vi "TBQ_AddPoint.vi"(9 "New Data Point":dbl, 11 "TimeBasedQueue In":refnum<class "TimeBasedQueue.lvclass">) -> (3 "TimeBasedQueue Out":refnum<class "TimeBasedQueue.lvclass">)   [LabVIEW 2012, in "TimeBasedQueue.lvclass"]
uses:
  TimeBasedQueue.lvclass
  TimeBasedQueue.lvclass/TimeBasedQueue.ctl
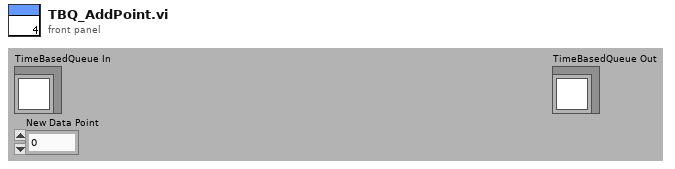
[diagram p1: front panel]
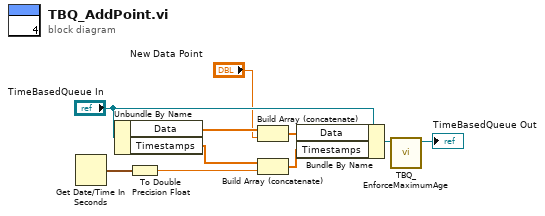
[diagram p0: block diagram]
diagram:
  n1 = Get Date/Time In Seconds() -> (seconds since 1Jan1904=w10:timestamp)
  n2 = Unbundle By Name("TimeBasedQueue In") -> ("Data"=w7:dbl[], "Timestamps"=w8:dbl[])
  n3 = To Double Precision Float(number=w10) -> (double precision float=w9:dbl)
  n4 = Build Array (concatenate)(w7, "New Data Point") -> (w1:dbl[])
  n5 = Build Array (concatenate)(w8, w9) -> (w6:dbl[])
  n6 = Bundle By Name(cluster="TimeBasedQueue In", "Data"=w1, "Timestamps"=w6) -> (w4:refnum<class "TimeBasedQueue.lvclass">)
  n7 = call "TBQ_EnforceMaximumAge.vi"("TimeBasedQueue In"=w4) -> ("TimeBasedQueue Out"=→"TimeBasedQueue Out":refnum<class "TimeBasedQueue.lvclass">)  [unwired: 10 in]
